vi "UpdateInertialData.vi"(11 "Update frequency":dbl) -> ()   [LabVIEW 2014]
uses:
  Variables/Physical data.vi
  Variables/Default global.vi
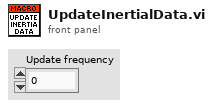
[diagram p1: front panel]
types:
  T1 = typedef "NI_Matrix.lvlib/RealMatrix.ctl" = dbl[][]
  T2 = cluster{"All Pod State Data":cluster{"Drive":cluster{"Drive Motor Output":dbl, "Wheel RPM":dbl, "Linear speed":dbl, "Linear acceleration":dbl, "Encoder Output":dbl, "Vmot":dbl, "Imot":dbl, "Torque":dbl, "Angular Momentum":dbl}, "Turret":cluster{"Turret Motor Output":dbl, "Turret Angle":dbl, "Turret velocity":dbl, "Turret acceleration":dbl, "Encoder Output":dbl, "Vmot":dbl, "Imot":dbl, "Torque":dbl, "Angular Momentum":dbl}, "Pod position (RCS)":cluster{"X":dbl, "Y":dbl, "Z":dbl}}[], "Global Robot Data":cluster{"Position Data":cluster{"Robot Position":cluster{"X":dbl, "Y":dbl, "Z":dbl}, "Robot Velocity":cluster{"X":dbl, "Y":dbl, "Z":dbl}, "Robot Acceleration":cluster{"X":dbl, "Y":dbl, "Z":dbl}}, "Rotation Data":cluster{"Angular Position":cluster{"X":dbl, "Y":dbl, "Z":dbl}, "Angular Velocity":cluster{"X":dbl, "Y":dbl, "Z":dbl}, "Angular Acceleration":cluster{"X":dbl, "Y":dbl, "Z":dbl}}}, "Inertial Characteristics":cluster{"Center of Mass (RCS)":cluster{"X":dbl, "Y":dbl, "Z":dbl}, "Mass Elements":cluster{"X":dbl, "Y":dbl, "Z":dbl, "Mass":dbl, "Name":string}[], "Center of Rotation (RCS)":cluster{"X":dbl, "Y":dbl, "Z":dbl}, "Tensor of Inertia":T1}}
  T3 = cluster{"X":dbl, "Y":dbl, "Z":dbl, "Mass":dbl, "Name":string}[]
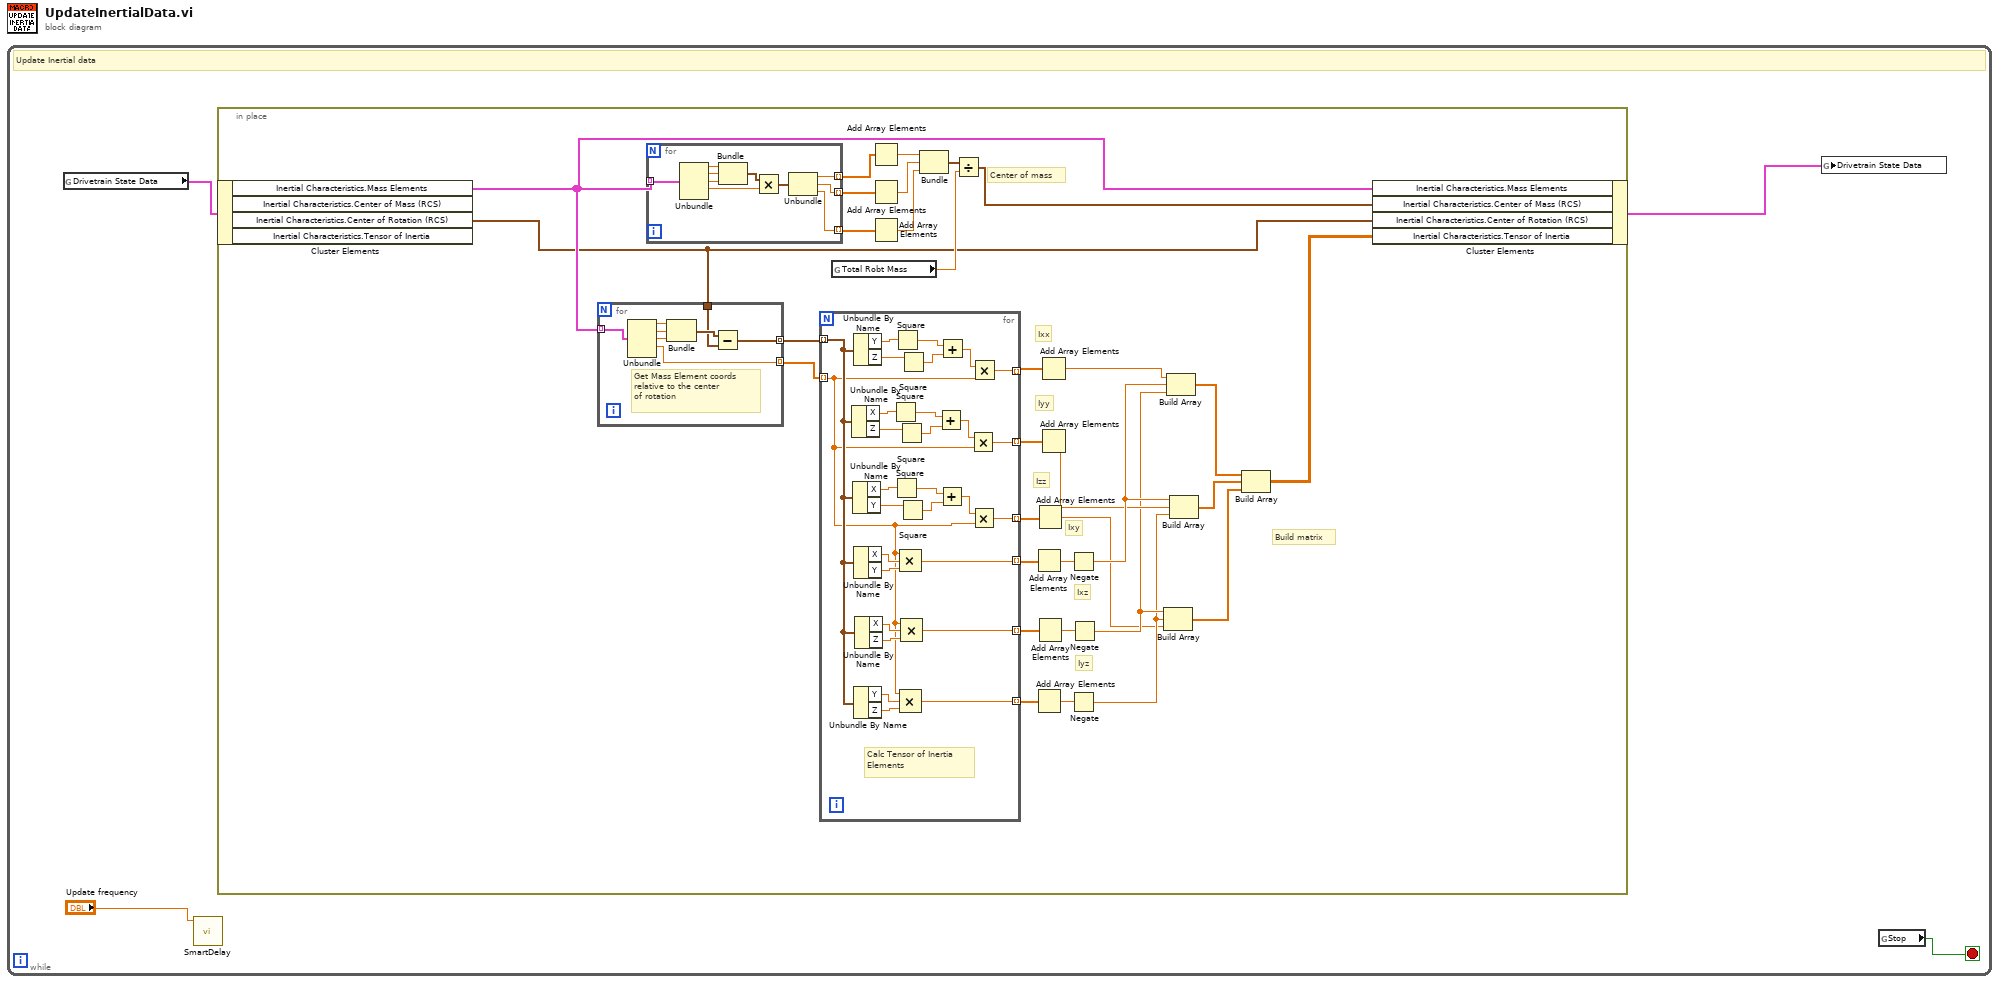
[diagram p0: block diagram]
diagram:
  n1 = while {
    stop <- w1 stop-if-true
    # "Update Inertial data"
    n2 = global read "Physical data.vi" "Drivetrain State Data"() -> (w4:T2)
    n3 = call "SmartDelay.vi"("Frequency"="Update frequency") -> ()  [unwired: 11 in]
    n4 = in-place {
      # "Build matrix"
      # "Iyz"
      # "Ixz"
      # "Ixy"
      # "Izz"
      # "Iyy"
      # "Ixx"
      # "Center of mass"
      n5 = in-place-cluster #1(w4) -> ("Inertial Characteristics.Mass Elements"=w24:T3, "Inertial Characteristics.Center of Rotation (RCS)"=w5:cluster{"X":dbl, "Y":dbl, "Z":dbl})  [unwired: 2 out]
      n6 = for {
        tunnel: w24 -> [w41] mode=indexing
        tunnel: w5 -> [w39]
        tunnel: [w38] -> w23 mode=indexing
        tunnel: [w37] -> w22 mode=indexing
        # "Get Mass Element coords\nrelative to the center\nof rotation"
        n7 = Unbundle(w41) -> ("X"=w42:dbl, "Y"=w44:dbl, "Z"=w43:dbl, "Mass"=w37:dbl)  [unwired: 1 out]
        n8 = Bundle("X"=w42, "Y"=w44, "Z"=w43) -> (w40:cluster{"X":dbl, "Y":dbl, "Z":dbl})  [unwired: 1 in]
        n9 = Subtract(x=w40, y=w39) -> (x-y=w38:cluster{"X":dbl, "Y":dbl, "Z":dbl})
      }
      n10 = for {
        tunnel: w24 -> [w83] mode=indexing
        tunnel: [w76] -> w31 mode=indexing
        tunnel: [w75] -> w30 mode=indexing
        tunnel: [w74] -> w29 mode=indexing
        n11 = Unbundle(w83) -> ("X"=w82:dbl, "Y"=w80:dbl, "Z"=w81:dbl, "Mass"=w79:dbl)  [unwired: 1 out]
        n12 = Bundle("X"=w82, "Y"=w80, "Z"=w81) -> (w78:cluster{"X":dbl, "Y":dbl, "Z":dbl})  [unwired: 1 in]
        n13 = Multiply(x=w78, y=w79) -> (x*y=w77:cluster{"X":dbl, "Y":dbl, "Z":dbl})
        n14 = Unbundle(w77) -> ("X"=w76:dbl, "Y"=w75:dbl, "Z"=w74:dbl)
      }
      n15 = for {
        tunnel: w23 -> [w46] mode=indexing
        tunnel: [w69] -> w27 mode=indexing
        tunnel: [w62] -> w26 mode=indexing
        tunnel: [w56] -> w25 mode=indexing
        tunnel: w22 -> [w45] mode=indexing
        tunnel: [w53] -> w21 mode=indexing
        tunnel: [w52] -> w18 mode=indexing
        tunnel: [w47] -> w17 mode=indexing
        # "Calc Tensor of Inertia\nElements"
        n16 = Unbundle By Name(w46) -> ("X"=w63:dbl, "Z"=w64:dbl)
        n17 = Unbundle By Name(w46) -> ("X"=w61:dbl, "Y"=w60:dbl)
        n18 = Unbundle By Name(w46) -> ("Y"=w73:dbl, "Z"=w72:dbl)
        n19 = Unbundle By Name(w46) -> ("X"=w54:dbl, "Y"=w55:dbl)
        n20 = Unbundle By Name(w46) -> ("Y"=w48:dbl, "Z"=w49:dbl)
        n21 = Unbundle By Name(w46) -> ("X"=w51:dbl, "Z"=w50:dbl)
        n22 = Square(x=w63) -> (x^2=w65:dbl)
        n23 = Square(x=w61) -> (x^2=w59:dbl)
        n24 = Square(x=w73) -> (x^2=w71:dbl)
        n25 = Square(x=w64) -> (x^2=w67:dbl)
        n26 = Square(x=w60) -> (x^2=w57:dbl)
        n27 = Square(x=w72) -> (x^2=w68:dbl)
        n28 = Compound Arithmetic op=MULTIPLY(w45, w54, w55) -> (w53:dbl)
        n29 = Compound Arithmetic op=MULTIPLY(w45, w48, w49) -> (w47:dbl)
        n30 = Compound Arithmetic op=MULTIPLY(w45, w51, w50) -> (w52:dbl)
        n31 = Add(x=w65, y=w67) -> (x+y=w66:dbl)
        n32 = Add(x=w59, y=w57) -> (x+y=w58:dbl)
        n33 = Add(x=w71, y=w68) -> (x+y=w70:dbl)
        n34 = Multiply(x=w66, y=w45) -> (x*y=w62:dbl)
        n35 = Multiply(x=w58, y=w45) -> (x*y=w56:dbl)
        n36 = Multiply(x=w70, y=w45) -> (x*y=w69:dbl)
      }
      n37 = global read "Physical data.vi" "Total Robt Mass"() -> (w33:dbl)
      n38 = Add Array Elements(numeric array=w31) -> (sum=w36:dbl)
      n39 = Add Array Elements(numeric array=w30) -> (sum=w35:dbl)
      n40 = Add Array Elements(numeric array=w29) -> (sum=w34:dbl)
      n41 = Bundle("X"=w36, "Y"=w35, "Z"=w34) -> (w32:cluster{"X":dbl, "Y":dbl, "Z":dbl})  [unwired: 1 in]
      n42 = Divide(x=w32, y=w33) -> (x/y=w28:cluster{"X":dbl, "Y":dbl, "Z":dbl})
      n43 = Add Array Elements(numeric array=w21) -> (sum=w20:dbl)
      n44 = Add Array Elements(numeric array=w17) -> (sum=w16:dbl)
      n45 = Add Array Elements(numeric array=w25) -> (sum=w10:dbl)
      n46 = Add Array Elements(numeric array=w18) -> (sum=w19:dbl)
      n47 = Add Array Elements(numeric array=w27) -> (sum=w15:dbl)
      n48 = Add Array Elements(numeric array=w26) -> (sum=w13:dbl)
      n49 = Negate(x=w20) -> (-x=w14:dbl)
      n50 = Negate(x=w16) -> (-x=w11:dbl)
      n51 = Negate(x=w19) -> (-x=w12:dbl)
      n52 = Build Array(w12, w11, w10) -> (w7:dbl[])
      n53 = Build Array(w15, w14, w12) -> (w9:dbl[])
      n54 = Build Array(w14, w13, w11) -> (w8:dbl[])
      n55 = Build Array(w9, w8, w7) -> (w6:dbl[][])
      n56 = in-place-cluster #1("Inertial Characteristics.Mass Elements"=w24, "Inertial Characteristics.Center of Mass (RCS)"=w28, "Inertial Characteristics.Center of Rotation (RCS)"=w5, "Inertial Characteristics.Tensor of Inertia"=w6) -> (w3:T2)
    }
    n57 = global write "Physical data.vi" "Drivetrain State Data"(w3) -> ()
    n58 = global read "Default global.vi" "Stop"() -> (w1:bool)
  }
